vi "Asylum_Driver_PreObjectInitialize.vi"(4 "Abort Notifier":refnum<notifier>, 8 "error in (no error)":errorcluster, 9 "Offsets":cluster{"X":dbl, "Y":dbl}, 10 "Pattern Data":T2, 11 "Application In":refnum<k7>) -> (0 "error out":errorcluster, 3 "Application Out":refnum<k7>)   [LabVIEW 2019]
uses:
  <userlib>/LevyLab/Relay Box/Typedefs/Resistor--enum.ctl
  <userlib>/LevyLab/Relay Box/Relay-Box.lvclass
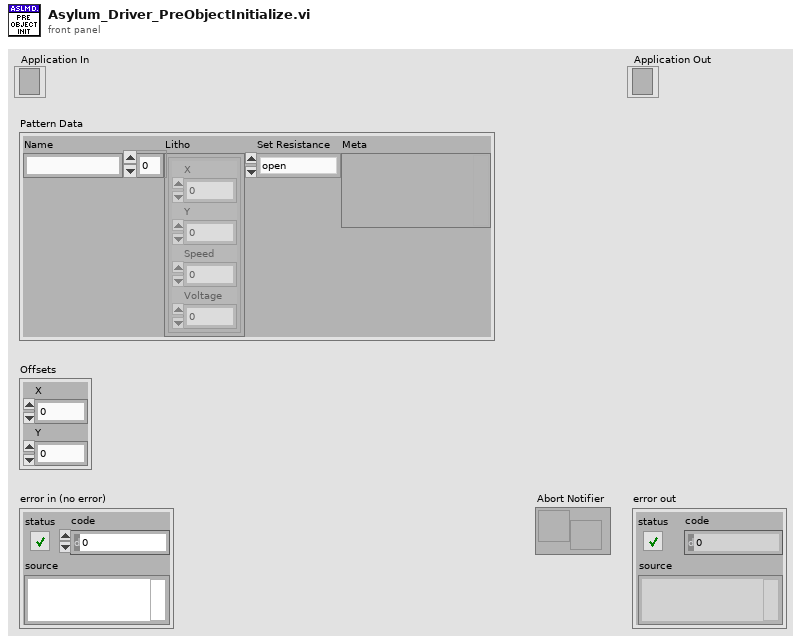
[diagram p1: front panel]
types:
  T1 = typedef "Relay-Box.lvclass/Resistor--enum.ctl" = enum16{"open", "discharge tip", "0 ohms", "100k ohm", "10M ohm", "1G ohm"}
  T2 = cluster{"Name":string, "Litho":cluster{"X":dbl, "Y":dbl, "Speed":dbl, "Voltage":dbl}[], "Set Resistance":T1, "Meta":variant}
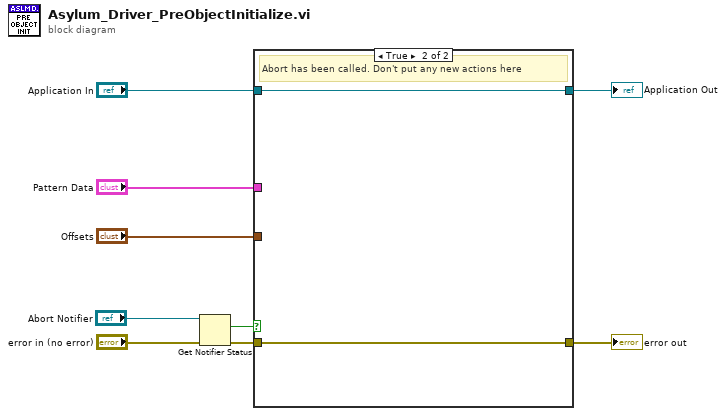
[diagram p0: block diagram]
diagram:
  n1 = Get Notifier Status(notifier="Abort Notifier", error in (no error)="error in (no error)") -> (current notification=w7:bool, error out=w6:errorcluster)  [unwired: 3 out]
  n2 = case shown="True" w7 {
    tunnel: w6 -> [w10 w13]
    tunnel: [w10 w13] -> w5
    tunnel: [w11 w12] -> w4
    tunnel: "Application In" -> [w11 w12]
    tunnel: "Pattern Data" -> [_ _]
    tunnel: "Offsets" -> [_ _]
    frame False {
    }
    frame True {
      # "Abort has been called. Don't put any new actions here"
    }
  }
  "error out" <- w5
  "Application Out" <- w4
